vi "Log Data Waveform.vi"(0 "TDMS Log In":refnum<class "TDMS Logger.lvclass">, 5 "Group Name":string, 7 "Channels Names":string[](array[string]), 9 "Data":waveform(dbl)[](array[waveform]), 11 "Error In":errorcluster) -> (4 "TDMS Log Out":refnum<class "TDMS Logger.lvclass">, 15 "Error Out":errorcluster)   [LabVIEW 2019, in "TDMS Logger.lvlib" / "TDMS Logger.lvclass"]
doc: "Send Waveform data to asynch logger."
uses:
  TDMS Logger.lvclass
  TDMS Logger.lvclass/TDMS Logger.ctl
  _Typedefs/Data Type.ctl
  _Typedefs/Log Message.ctl
  _Typedefs/Log Action.ctl
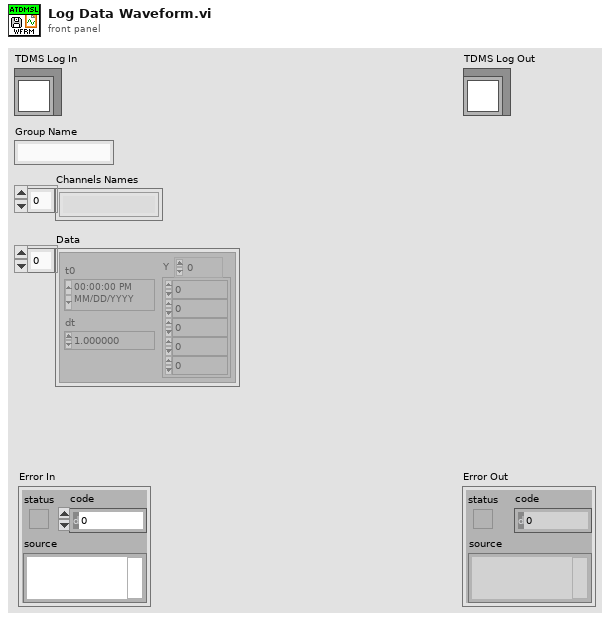
[diagram p1: front panel]
types:
  T1 = typedef "TDMS Logger.lvlib/TDMS Logger.lvclass/Data Type.ctl" = enum16{"I16", "I8", "String", "U16", "U8", "Waveform", "Double", "Single"}
  T2 = typedef "TDMS Logger.lvlib/TDMS Logger.lvclass/Log Message.ctl" = cluster{"Log Action":T3, "Variant":variant, "Data Type":T1, "Group Name":string, "Channels Names":string[]}
  T3 = typedef "TDMS Logger.lvlib/TDMS Logger.lvclass/Log Action.ctl" = enum16{"Handle Old Files", "Status Update", "Stop", "Log Data", "Initialize"}
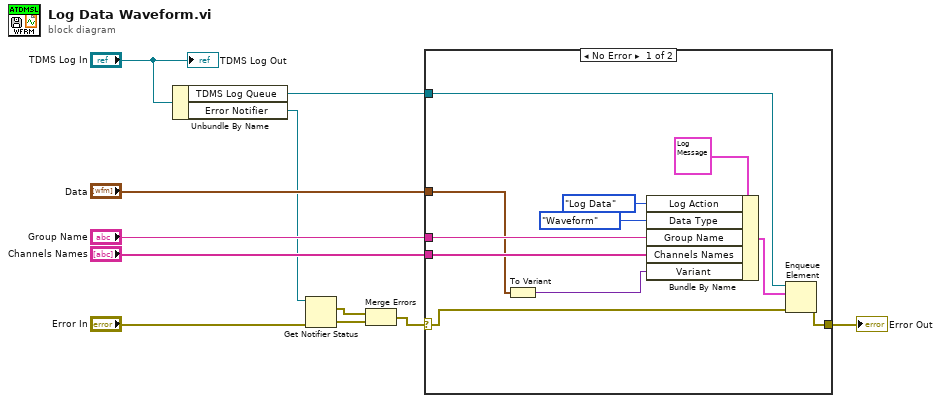
[diagram p0: block diagram]
diagram:
  n1 = Unbundle By Name("TDMS Log In") -> ("TDMS Log Queue"=w7:refnum<queue>, "Error Notifier"=w4:refnum<notifier>)
  n2 = Get Notifier Status(notifier=w4, error in (no error)="Error In") -> (current notification=w1:errorcluster, error out=w2:errorcluster)  [unwired: 3 out]
  n3 = Merge Errors(w1, w2) -> (w3:errorcluster)
  n4 = case shown="No Error" w3 {
    selector: w3 -> [w15 w23]
    tunnel: [w14 w23] -> w11
    tunnel: "Group Name" -> [w18 _]
    tunnel: "Channels Names" -> [w17 _]
    tunnel: "Data" -> [w13 _]
    tunnel: w7 -> [w16 _]
    frame No Error {
      n5 = To Variant(anything=w13) -> (Variant=w12:variant)
      n6 = Bundle By Name(cluster=T2 {"Log Action"=enum."Stop", "Variant"=variant, "Data Type"=enum."String", "Group Name"="", "Channels Names"=[]} ("element"), "Log Action"=Log_Action."Log Data", "Data Type"=Data_Type."Waveform", "Group Name"=w18, "Channels Names"=w17, "Variant"=w12) -> (w21:T2)
      n7 = Enqueue Element(queue=w16, element=w21, error in (no error)=w15) -> (error out=w14:errorcluster)  [unwired: 1 in, 2 out]
    }
    frame Error {
    }
  }
  "Error Out" <- w11
  "TDMS Log Out" <- "TDMS Log In"
